vi "ScaniValve_client.vi"(0 "Port Number":u8=1 max=47 step=1) -> (1 "Achieved Posn.":T1=8 max=23 step=1, 2 "Diverter Valve":bool, 3 "Error String":string)   [LabVIEW 2010]
uses:
  Anemometry/Anemometry Sub Vis/Baratron Scanning Valve/scanning_valve_tl.ctl
  ADAM Server/Sub VI's/Channel_Description_Global.vi
  Anemometry/Anemometry Sub Vis/Globals/Preference_global.vi
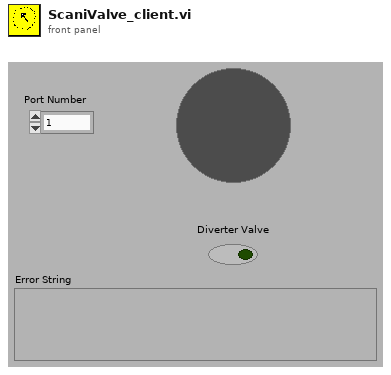
[diagram p1: front panel]
types:
  T1 = typedef "scanning_valve_tl.ctl" = u8
  T2 = enum16{"Load ADAM setup from excel file", "Save ADAM setup to excel file"}
  T3 = typedef "Ch_description_ADAM.ctl" = cluster{"Ch Name":string, "Type":T4, "Function":T5, "Ch State":T6, "Calibration type":T7, "A":dbl, "B":dbl, "C":dbl, "D":dbl, "Comments":string, "Address":T8, "String":string, "Duty":u16}
  T4 = typedef "Module_type_ADAM.ctl" = enum16{"4011", "4012", "4013", "4014", "4016", "4017", "4018", "4021", "4050", "4052", "4053", "4060", "4080", "5000", "5017", "5018", "5024", "5051", "5056", "5060", "6060", "Tracker", "WEST", "GILL", "JEM", "VICI", "Vaisala", "DRUCK", "Run VI Named:", "IR2100", "PPT", "Comparator", "VIRTUAL", "Hold Value", "Read A", "Read Ch", "Coded", "Client Info", "Web Client", "X10", "Test"}
  T5 = typedef "Function_ADAM.ctl" = enum16{"Analogue Input", "Digital Input", "Event counter", "Event rate", "Analogue Output", "Digital Output", "Relay Output"}
  T6 = typedef "Channel_State.ctl" = enum16{"On", "Off", "Always On", "Always Off"}
  T7 = typedef "Calib_type_ADAM.ctl" = enum16{"Raw", "Bx + A", "Cx^2 + Bx + A", "Dx^3 + Cx^2 + Bx + A", "In Band", "Hi-Tec Q", "Hi-Tec M_dot", "Text"}
  T8 = typedef "Address.ctl" = cluster{"Main":i32, "Ch.":i32, "Sub":i32, "Port Name":string}
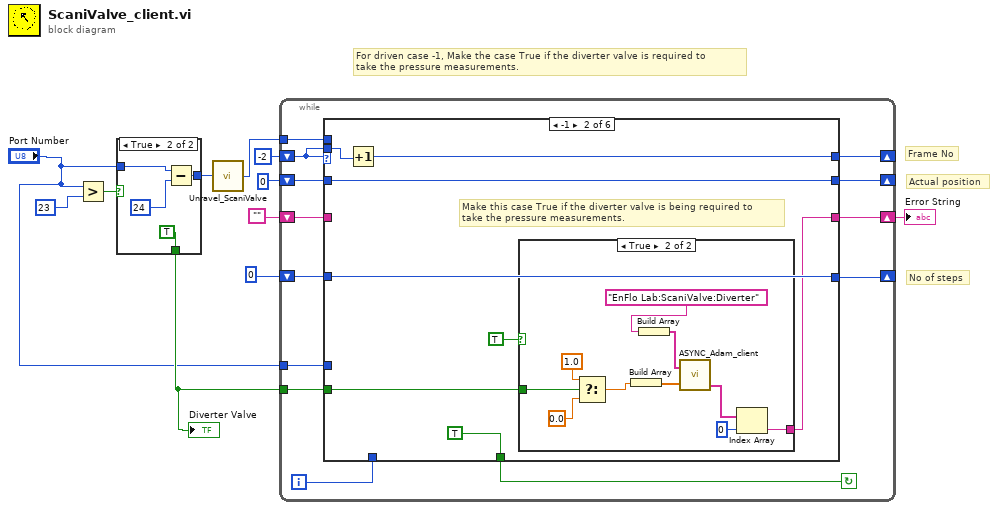
[diagram p0: block diagram]
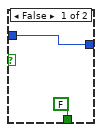
[diagram p2: hidden frame]
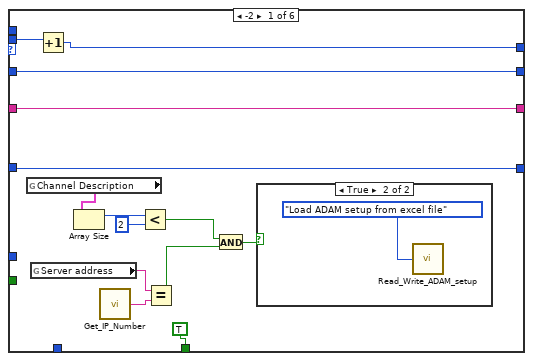
[diagram p3: hidden frame]
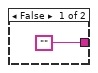
[diagram p5: hidden frame]
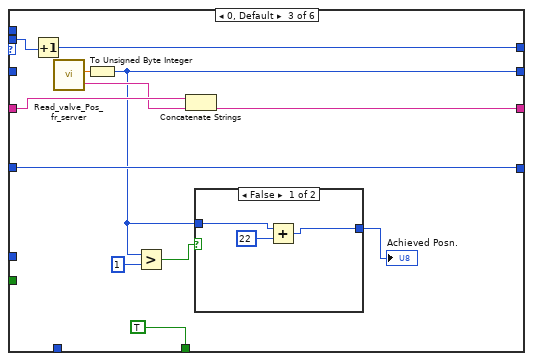
[diagram p6: hidden frame]
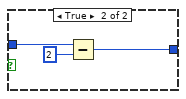
[diagram p7: hidden frame]
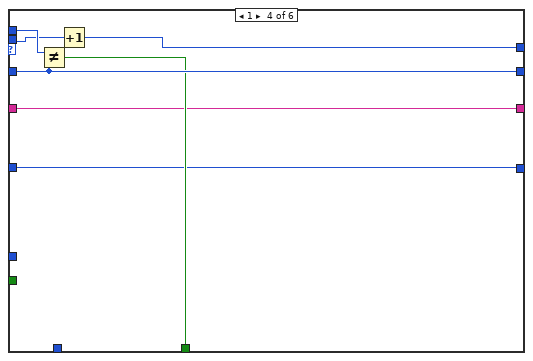
[diagram p8: hidden frame]
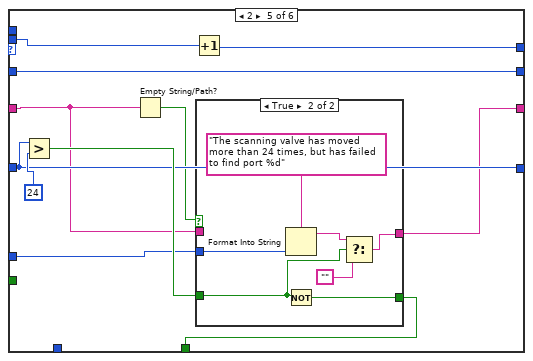
[diagram p9: hidden frame]
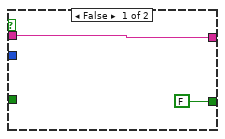
[diagram p10: hidden frame]
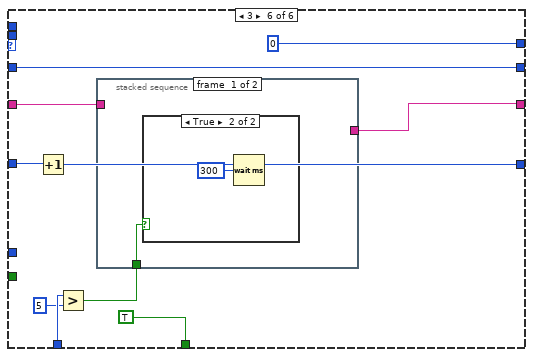
[diagram p11: hidden frame]
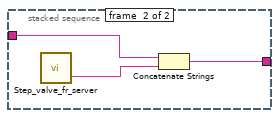
[diagram p13: hidden frame]
diagram:
  # "For driven case -1, Make the case True if the diverter valve is required to \ntake the pressure measurements."
  # "No of steps"
  # "Actual position"
  # "Frame No"
  n1 = Greater?(x="Port Number", y=u8 23) -> (0:w7:bool)
  n2 = case shown="True" w7 {
    tunnel: [FALSE TRUE] -> w6
    tunnel: "Port Number" -> [w12 w16]
    tunnel: [w12 w15] -> w2
    frame False {
    }
    frame True {
      n3 = Subtract(x=w16, y=u8 24) -> (x-y=w15:u8)
    }
  }
  "Diverter Valve" <- w6
  n4 = call "Unravel_ScaniValve.vi"("Port Number"=w2) -> ("Port Number out"=w1:u8)
  n5 = while {
    shift-left: "" -> [w21]
    shift-right: [w22] -> w4
    tunnel: w1 -> [w24]
    shift-left: 0 -> [w26]
    shift-right: [w25] -> _
    shift-left: u8 0 ("Valve Position") -> [w28]
    shift-right: [w29] -> _
    shift-left: -2 -> [w23]
    shift-right: [w30] -> _
    tunnel: w6 -> [w20]
    tunnel: "Port Number" -> [w19]
    i -> [w18]
    stop <- w27 continue-if-true
    n6 = case shown="-1" w23 {
      tunnel: [w43 w53 w76 w85 w97 0] -> w30
      tunnel: [w42 w47 w66 w88 w96 w119] -> w29
      tunnel: w28 -> [w42 w47 _ w88 w96 w119]
      tunnel: w24 -> [_ _ _ w89 _ _]
      tunnel: [TRUE TRUE TRUE w87 w90 TRUE] -> w27
      tunnel: w26 -> [w33 w51 w74 w86 w98 w117]
      tunnel: [w33 w51 w74 w86 w98 w116] -> w25
      tunnel: w23 -> [w44 w50 w72 w84 w95 _]
      tunnel: [w34 w48 w69 w83 w93 w113] -> w22
      tunnel: w21 -> [w34 _ w71 w83 w94 w114]
      tunnel: w20 -> [_ w49 _ _ _ _]
      tunnel: w19 -> [_ _ _ _ w92 _]
      tunnel: w18 -> [_ _ _ _ _ w112]
      frame -2 {
        n7 = global read "Channel_Description_Global.vi" "Channel Description"() -> (w39:T3[])
        n8 = global read "Preference_global.vi" "Server address"() -> (w40:string)
        n9 = Increment(x=w44) -> (x+1=w43:i32)
        n10 = Array Size(array=w39) -> (size(s)=w38:i32)
        n11 = call "Get_IP_Number.vi"() -> ("IP Number"=w41:string)
        n12 = Less?(x=w38, y=2) -> (x < y?=w32:bool)
        n13 = Equal?(x=w40, y=w41) -> (x = y?=w36:bool)
        n14 = And(x=w32, y=w36) -> (x .and. y?=w35:bool)
        n15 = case shown="True" w35 {
          frame False {
          }
          frame True {
            n16 = call "Read_Write_ADAM_setup.vi"("Mode"=T2."Load ADAM setup from excel file") -> ()  [unwired: 4 out]
          }
        }
      }
      frame -1 {
        # "Make this case True if the diverter valve is being required to \ntake the pressure measurements."
        n17 = Increment(x=w50) -> (x+1=w53:i32)
        n18 = case shown="True" TRUE {
          tunnel: w49 -> [_ w56]
          tunnel: ["" w55] -> w48
          frame False {
          }
          frame True {
            n19 = Select(t=1.0, s=w56, f=0.0) -> (s? t:f=w59:dbl)
            n20 = Build Array(w59) -> (w60:dbl[])
            n21 = Build Array("EnFlo Lab:ScaniValve:Diverter") -> (w57:string[])
            n22 = call "ASYNC_Adam_client.vi"("Values"=w60, "Channel Names"=w57) -> ("Scan Comments"=w61:string[])  [unwired: 1 out]
            n23 = Index Array(array=w61, index=0 ("Index")) -> (element=w55:string)
          }
        }
      }
      frame 0, Default {
        n24 = Increment(x=w72) -> (x+1=w76:i32)
        n25 = call "Read_valve_Pos_fr_server.vi"() -> ("Valve Error Info"=w70:string, "Output Value"=w73:dbl)  [unwired: 1 in, 1 out]
        n26 = To Unsigned Byte Integer(number=w73) -> (unsigned 8bit integer=w66:u8)
        n27 = Greater?(x=w66, y=u8 1) -> (0:w67:bool)
        n28 = Concatenate Strings(w71, w70) -> (w69:string)
        n29 = case shown="False" w67 {
          tunnel: w66 -> [w79 w82]
          tunnel: [w77 w80] -> w65
          frame False {
            n30 = Add(x=w79, y=u8 22) -> (x+y=w77:u8)
          }
          frame True {
            n31 = Subtract(x=w82, y=u8 2) -> (x-y=w80:u8)
          }
        }
        "Achieved Posn." <- w65
      }
      frame 1 {
        n32 = Not Equal?(x=w89, y=w88) -> (x != y?=w87:bool)
        n33 = Increment(x=w84) -> (x+1=w85:i32)
      }
      frame 2 {
        n34 = Greater?(x=w98, y=24) -> (0:w99:bool)
        n35 = Empty String/Path?(string/path=w94) -> (empty?=w91:bool)
        n36 = Increment(x=w95) -> (x+1=w97:i32)
        n37 = case shown="True" w91 {
          tunnel: w99 -> [_ w106]
          tunnel: w94 -> [w102 _]
          tunnel: w92 -> [_ w109]
          tunnel: [w102 w104] -> w93
          tunnel: [FALSE w107] -> w90
          frame False {
          }
          frame True {
            n38 = Format Into String(format string="The scanning valve has moved more than 24 times, but has failed to find port %d" ("Format String"), w109) -> (resulting string=w105:string)  [unwired: 2 in, 1 out]
            n39 = Not(x=w106) -> (.not. x?=w107:bool)
            n40 = Select(t=w105, s=w106, f="") -> (s? t:f=w104:string)
          }
        }
      }
      frame 3 {
        n41 = Increment(x=w117) -> (x+1=w116:i32)
        n42 = Greater?(x=w112, y=5) -> (0:w110:bool)
        n43 = stacked-sequence {
          tunnel: w114 -> [_ w123]
          tunnel: [_ w122] -> w113
          tunnel: w110 -> [w120 _]
          frame #0 {
            n44 = case shown="True" w120 {
              frame False {
              }
              frame True {
                n45 = Wait (ms)(milliseconds to wait=u32 300) -> ()  [unwired: 1 out]
              }
            }
          }
          frame #1 {
            n46 = call "Step_valve_fr_server.vi"() -> ("Valve Error Info"=w124:string)  [unwired: 3 out]
            n47 = Concatenate Strings(w123, w124) -> (w122:string)
          }
        }
      }
    }
  }
  "Error String" <- w4
